vi "simple_cache_bool.vi"(1 "refresh":bool, 2 "bool":bool) -> (0 "$_val":bool)   [LabVIEW 2018]
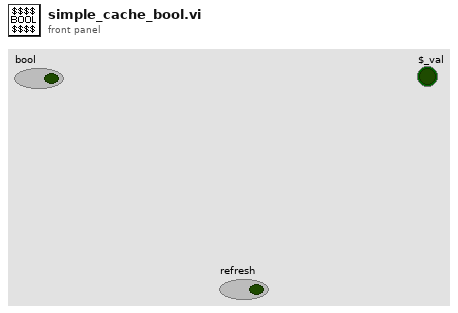
[diagram p1: front panel]
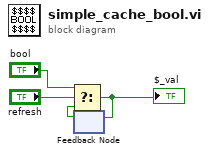
[diagram p0: block diagram]
diagram:
  n1 = feedback #1() -> (w2:bool)  [unwired: 1 in]
  n2 = Select(t="bool", s="refresh", f=w2) -> (s? t:f=w3:bool)
  "$_val" <- w3
  n3 = feedback-in #1(w3) -> ()
